vi "BestAttackLocations.vi"(1 "AttackMap DVR":T1) -> (0 "Locations":T2[](array[typedef]))   [LabVIEW 2020, in "Atom.lvclass"]
uses:
  Atom.lvclass
  Common/Position.ctl
  AttackMap DVR.ctl
  Common/Common.lvlib
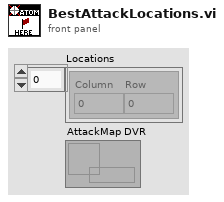
[diagram p1: front panel]
types:
  T1 = typedef "Atom.lvclass/AttackMap DVR.ctl" = refnum<data-value>
  T2 = typedef "Common.lvlib/Position.ctl" = cluster{"Column":i32, "Row":i32}
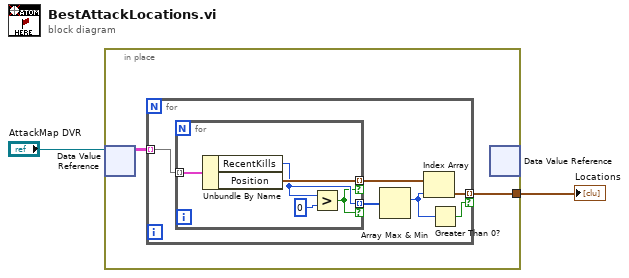
[diagram p0: block diagram]
diagram:
  n1 = in-place {
    in-place-border: [w3] -> w1
    n2 = in-place-dvr #1("AttackMap DVR") -> (w4:cluster{"RecentKills":i32, "Position":T2}[][])  [unwired: 1 out]
    n3 = for {
      tunnel: w4 -> [w10] mode=indexing
      tunnel: [w7] -> w3 mode=indexing if=w5
      n4 = for {
        tunnel: w10 -> [w15] mode=indexing
        tunnel: [w13] -> w9 mode=indexing if=w12
        tunnel: [w14] -> w8 mode=indexing if=w12
        n5 = Unbundle By Name(w15) -> ("RecentKills"=w13:i32, "Position"=w14:T2)
        n6 = Greater?(x=w13, y=0) -> (0:w12:bool)
      }
      n7 = Array Max & Min(array=w9) -> (max index (indices)=w6:i32)  [unwired: 3 out]
      n8 = Index Array(array=w8, index=w6) -> (element=w7:T2)
      n9 = Greater Than 0?(x=w6) -> (x > 0?=w5:bool)
    }
    n10 = in-place-dvr #1() -> ()  [unwired: 1 in, 2 out]
  }
  "Locations" <- w1
